vi "mqttClient_ModelController.vi"() -> ()   [LabVIEW 2019]
uses:
  state -- cluster.ctl
  <vilib>/LabVIEW Open Source Project/OpenSerializer JKI JSON/Serializer.JSON.lvclass
  C:/Program Files (x86)/National Instruments/LabVIEW 2019/vi.lib/LabVIEW Open Source Project/OpenSerializer/Serializer/Serializer.lvclass
  target -- cluster.ctl
  <vilib>/LabVIEW Open Source Project/MQTT Connection/MQTT_Base/Base Class/MQTT_Base.lvclass/MQTT_Base.ctl
  <vilib>/LabVIEW Open Source Project/MQTT Client/Client class/Client.lvclass/Client.ctl
  <vilib>/LabVIEW Open Source Project/MQTT Control Packets/Control Packets/ControlPacket/QualityOfService -- enum.ctl
  <vilib>/LabVIEW Open Source Project/MQTT Control Packets/Control Packets/ControlPacket/ControlPacket.lvclass/ControlPacket.ctl
  <vilib>/LabVIEW Open Source Project/MQTT Control Packets/Control Packets/CONNECT/ConnectFlags -- cluster.ctl
  <vilib>/LabVIEW Open Source Project/MQTT TCP Connection/MQTT_TCP/Connection/TCPConnection.lvclass
  C:/Program Files (x86)/National Instruments/LabVIEW 2019/vi.lib/LabVIEW Open Source Project/MQTT Connection/MQTT_Connection/Connection/Connection.lvclass
  <vilib>/LabVIEW Open Source Project/MQTT Client/Client class/Client.lvclass
  C:/Program Files (x86)/National Instruments/LabVIEW 2019/vi.lib/LabVIEW Open Source Project/MQTT Connection/MQTT_Base/Base Class/MQTT_Base.lvclass
  <vilib>/LabVIEW Open Source Project/OpenSerializer/Serializer.FlattenedString/Serializer.FlattenedString.lvclass
  <vilib>/LabVIEW Open Source Project/MQTT Control Packets/Control Packets/PUBLISH/PUBLISH.lvclass
  C:/Program Files (x86)/National Instruments/LabVIEW 2019/vi.lib/LabVIEW Open Source Project/MQTT Control Packets/Control Packets/ControlPacket/ControlPacket.lvclass
  <vilib>/LabVIEW Open Source Project/OpenSerializer/Serializer/Serializer.lvclass
  <vilib>/numeric/Random Number (Range) DBL.vi
  <vilib>/LabVIEW Open Source Project/MQTT Connection/MQTT_Base/Base Class/MQTT_Base.lvclass
  <vilib>/LabVIEW Open Source Project/MQTT Control Packets/Control Packets/ControlPacket/ControlPacket.lvclass
  <vilib>/LabVIEW Open Source Project/MQTT Control Packets/Control Packets/CONNECT/CONNECT.lvclass
panel:
  in  "Connection":bool
  out "Last Error":errorcluster
  out "Incoming Payload":string
  out "state":T1 {"measured" format="%.1g"; "setpoint" format="%.1g"}
  # "Native LabVIEW MQTT Client (Model - Controller)"
  # "G Open Source Project for LabVIEW\nhttps://github.com/LabVIEW-Open-Source/MQTT-Client"
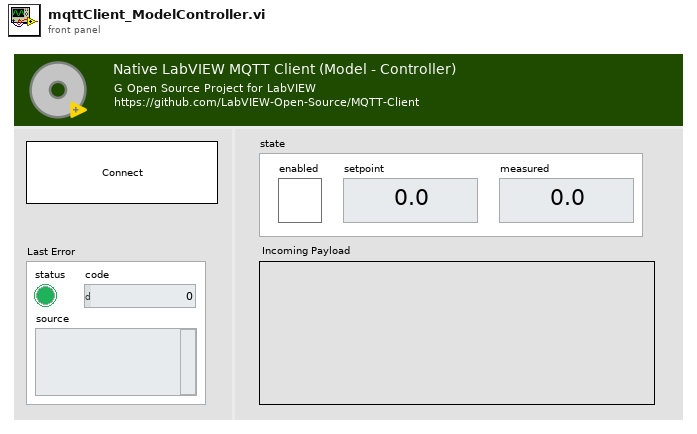
[diagram p1: front panel]
types:
  T1 = typedef "state -- cluster.ctl" = cluster{"enabled":bool, "setpoint":dbl, "measured":dbl}
  T2 = typedef "target -- cluster.ctl" = cluster{"enabled":bool, "setpoint":dbl, "responseURI":string}
  T3 = cluster{"appName":string, "state":T1, "target":T2}
  T4 = typedef "MQTT Client.lvlib/Client.lvclass/Public Events -- cluster.ctl" = cluster{"Connection Status":refnum<user-event>, "Connected":refnum<user-event>, "Application Message":refnum<user-event>}
  T5 = typedef "MQTT Base.lvlib/MQTT_Base.lvclass/Public Events -- cluster.ctl" = cluster{"Stop Event":refnum<user-event>, "Error Event":refnum<user-event>, "Inbound Message":refnum<user-event>}
  T6 = typedef "MQTT_Control_Packets.lvlib/ControlPacket.lvclass/QualityOfService -- enum.ctl" = enum16{"0 (At Most Once)", "1 (At Least Once)", "2 (Exactly Once)"}
  T7 = typedef "MQTT_Control_Packets.lvlib/CONNECT.lvclass/ConnectFlags -- cluster.ctl" = cluster{"Reserved":bool, "Clean Session":bool, "Will Flag":bool, "Will QoS 1":bool, "Will QoS 2":bool, "Will Retain":bool, "Password Flag":bool, "User Name Flag":bool}
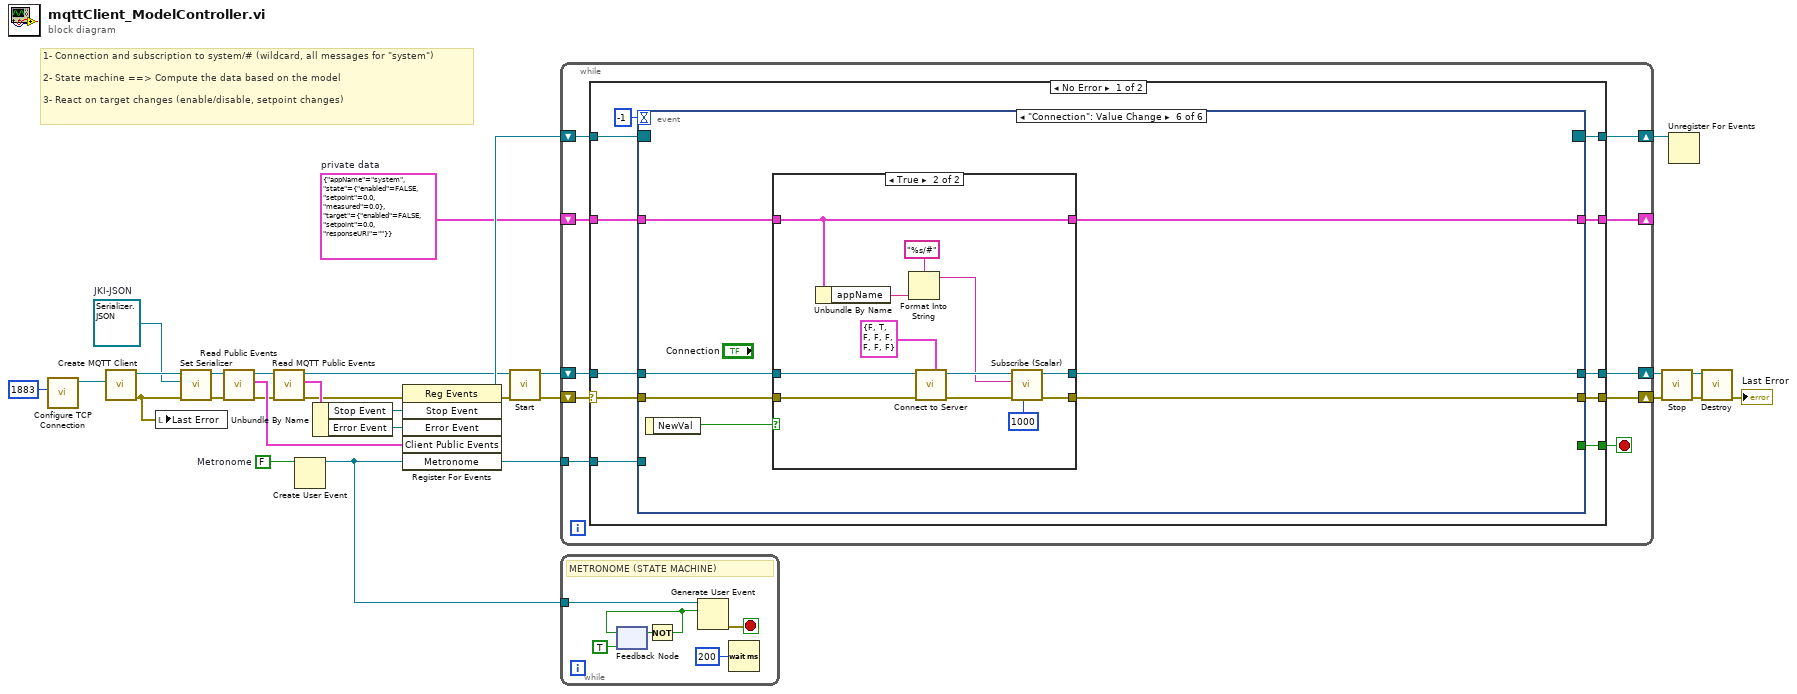
[diagram p0: block diagram]
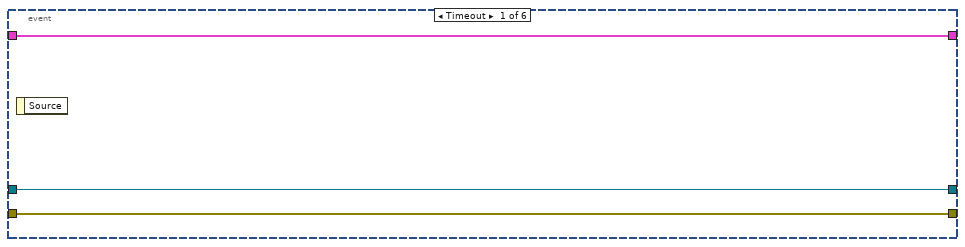
[diagram p2: hidden frame]
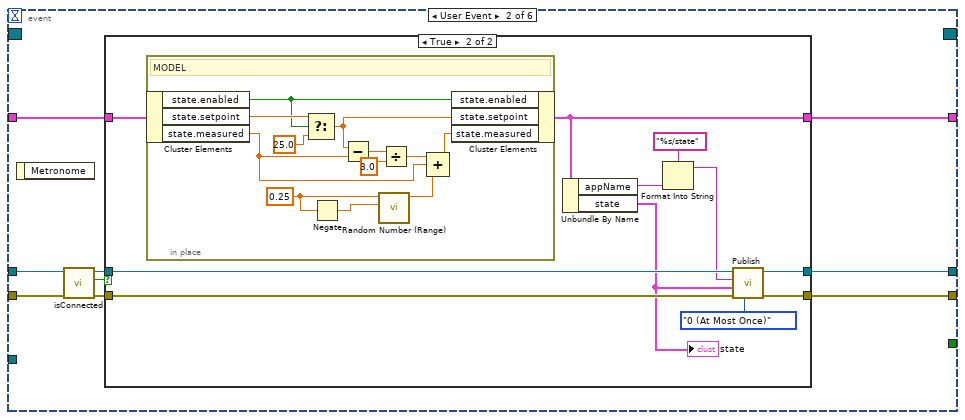
[diagram p3: hidden frame]
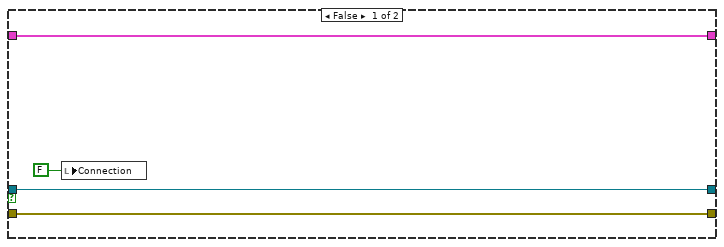
[diagram p4: hidden frame]
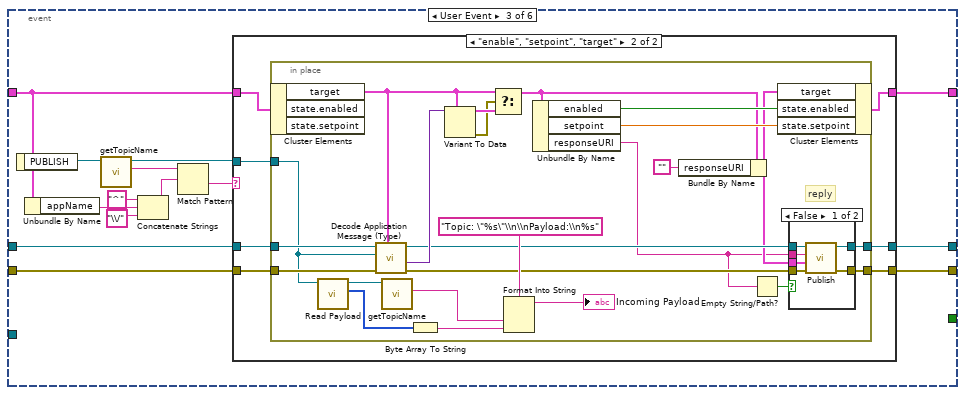
[diagram p5: hidden frame]
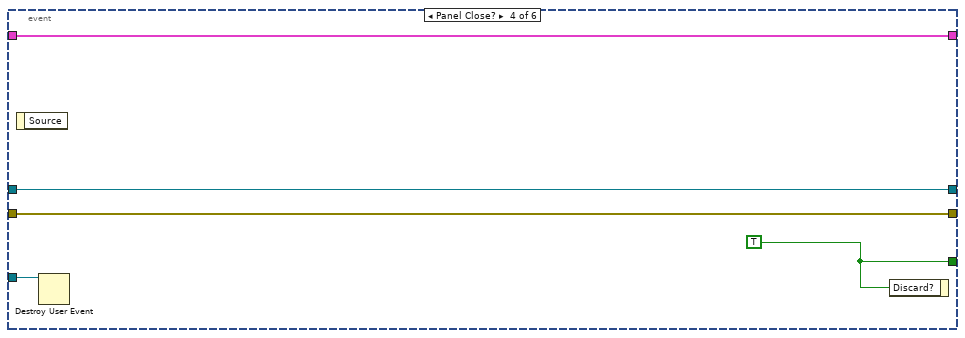
[diagram p8: hidden frame]
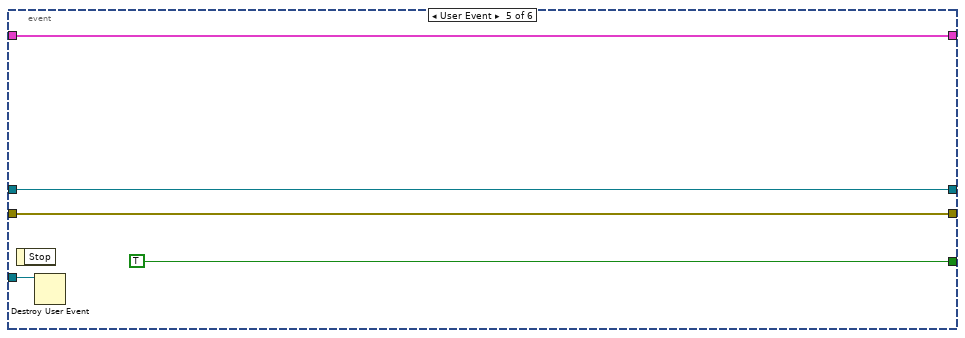
[diagram p9: hidden frame]
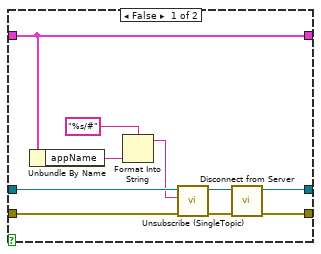
[diagram p10: hidden frame]
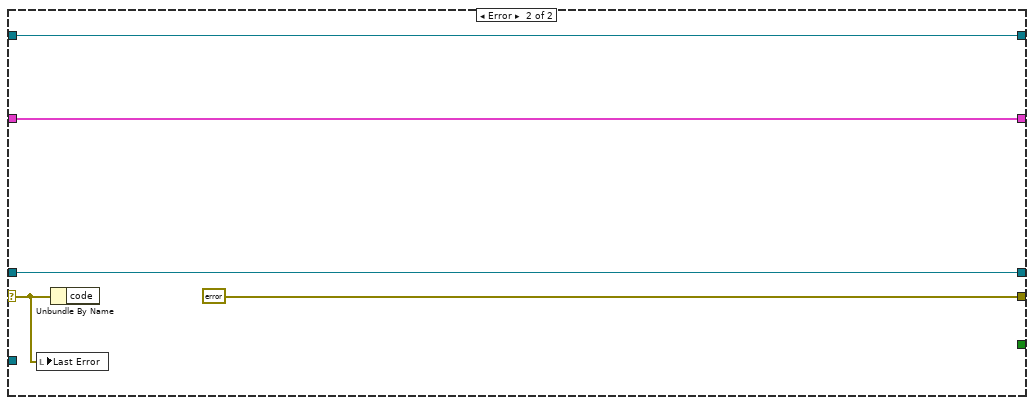
[diagram p11: hidden frame]
diagram:
  w2 = FALSE  # Metronome
  w4 = T3 {"appName"="system", "state"={"enabled"=FALSE, "setpoint"=0.0, "measured"=0.0}, "target"={"enabled"=FALSE, "setpoint"=0.0, "responseURI"=""}}  # private data
  w7 = refnum<class "Serializer.JSON.lvclass"> refnum  # JKI-JSON
  # "1- Connection and subscription to system/# (wildcard, all messages for \"system\")\n\n2- State machine ==> Compute the data based on the model\n\n3- React on target changes (enable/disable, setpoint changes)"
  n1 = call <vilib>:"Configure TCP Connection.vi"("remote port (80)"=u16 1883) -> ("TCPConnection"=w11:refnum<class "TCPConnection.lvclass">)  [unwired: 9 in, 1 out]
  n2 = call <vilib>:"Create MQTT Client.vi"("Connection Configuration"=w11) -> ("error out"=w3:errorcluster, "Client out"=w10:refnum<class "Client.lvclass">)  [unwired: 9 in]
  n3 = local write "Last Error"(w3) -> ()
  n4 = call <vilib>:"Set Serializer.vi"("error in (no error)"=w3, "Serializer (default: Flattened String)"=w7, "MQTT_Base"=w10) -> ("error out"=w8:errorcluster, "MQTT_Base out"=w9:refnum<class "Client.lvclass">)  [unwired: 7 in]
  n5 = call <vilib>:"Read Public Events.vi"("error in (no error)"=w8, "Client in"=w9) -> ("error out"=w13:errorcluster, "Client Public Events"=w15:T4, "Client out"=w12:refnum<class "Client.lvclass">)  [unwired: 7 in]
  n6 = call <vilib>:"Read MQTT Public Events.vi"("error in (no error)"=w13, "MQTT_Base in"=w12) -> ("error out"=w14:errorcluster, "MQTT Public Events"=w22:T5, "MQTT_Base out"=w17:refnum<class "Client.lvclass">)  [unwired: 7 in]
  n7 = Create User Event(user event datatype=w2) -> (user event=w1:refnum<user-event>)  [unwired: 1 in, 1 out]
  n8 = Unbundle By Name(w22) -> ("Stop Event"=w20:refnum<user-event>, "Error Event"=w21:refnum<user-event>)
  n9 = register-events(error in=w14, w20, w21, w15, w1) -> (reference out=w18:refnum<event-registration>, error out=w16:errorcluster)  [unwired: 1 in]
  n10 = call <vilib>:"Start.vi"("error in (no error)"=w16, "MQTT_Base in"=w17) -> ("error out"=w5:errorcluster, "MQTT_Base out"=w6:refnum<class "Client.lvclass">)  [unwired: 7 in, 1 out]
  n11 = while {
    shift-right: [w37] -> w19
    shift-left: w18 -> [w38]
    shift-right: [w34] -> w24
    shift-left: w6 -> [w35]
    shift-right: [w36] -> w26
    shift-left: w5 -> [w32]
    shift-right: [w30] -> _
    shift-left: w4 -> [w31]
    tunnel: w1 -> [w29]
    stop <- w33 stop-if-true
    n12 = case shown="No Error" w32 {
      selector: w32 -> [w42 w187]
      tunnel: w38 -> [w49 w186]
      tunnel: [w48 w186] -> w37
      tunnel: [w47 errorcluster {"status"=FALSE, "code"=0, "source"=""} ("error out")] -> w36
      tunnel: w35 -> [w45 w188]
      tunnel: [w44 w188] -> w34
      tunnel: [w43 _] -> w33
      tunnel: w31 -> [w41 w185]
      tunnel: [w40 w185] -> w30
      tunnel: w29 -> [w39 _]
      frame No Error {
        n13 = event shown="[5] \"Connection\": Value Change" {
          selector: w49 -> [_ _ _ _ _ _]
          dyn-events: [_ _ _ _ _ _] -> w48
          timeout: -1 -> [_ _ _ _ _ _]
          tunnel: w42 -> [w50 w57 w99 w147 w154 w157]
          tunnel: [w50 w60 w97 w147 w154 w158] -> w47
          tunnel: [_ _ _ w149 TRUE _] -> w43
          tunnel: w45 -> [w51 w59 w100 w148 w152 w161]
          tunnel: [w51 w61 w98 w148 w152 w159] -> w44
          tunnel: w41 -> [w52 w54 w95 w146 w151 w155]
          tunnel: [w52 w53 w96 w146 w151 w156] -> w40
          tunnel: w39 -> [_ _ _ w145 w150 _]
          event Timeout {
            n14 = event-data() -> ()  [unwired: 1 in, 1 out]
          }
          event User Event {
            n15 = event-data() -> ()  [unwired: 1 in, 1 out]
            n16 = call <vilib>:"isConnected.vi"("error in (no error)"=w57, "Client in"=w59) -> ("error out"=w56:errorcluster, "connected"=w55:bool, "Client out"=w58:refnum<class "Client.lvclass">)  [unwired: 7 in]
            n17 = case shown="True" w55 {
              tunnel: [w65 w75] -> w61
              tunnel: [w64 w73] -> w60
              tunnel: w58 -> [w65 w76]
              tunnel: w56 -> [w64 w74]
              tunnel: w54 -> [w62 w69]
              tunnel: [w62 w68] -> w53
              frame False {
                n18 = local write "Connection"(FALSE ("Connection")) -> ()
              }
              frame True {
                n19 = in-place {
                  w78 = 0.25 ("lower bound (0)")
                  # "MODEL"
                  n20 = in-place-cluster #1(w69) -> ("state.enabled"=w86:bool, "state.setpoint"=w87:dbl, "state.measured"=w81:dbl)
                  n21 = Select(t=w87, s=w86, f=25.0) -> (s? t:f=w85:dbl)
                  n22 = Negate(x=w78) -> (-x=w79:dbl)
                  n23 = Subtract(x=w85, y=w81) -> (x-y=w83:dbl)
                  n24 = call-poly <vilib>:"Random Number (Range).vi"("lower bound (0)"=w79, "upper bound (100)"=w78) -> ("number"=w77:dbl)  [unwired: 9 in]
                  n25 = Divide(x=w83, y=3.0 ("f")) -> (x/y=w82:dbl)
                  n26 = Compound Arithmetic op=ADD(w82, w81, w77) -> (w80:dbl)
                  n27 = in-place-cluster #1("state.enabled"=w86, "state.setpoint"=w85, "state.measured"=w80) -> (w68:T3)
                }
                n28 = Unbundle By Name(w68) -> ("appName"=w66:string, "state"=w67:T1)
                "state" <- w67
                n29 = Format Into String(format string="%s/state" ("Topic Name (empty: Payload name)"), w66) -> (resulting string=w70:string)  [unwired: 2 in, 1 out]
                n30 = call <vilib>:"Publish.vi"("QoS"=QualityOfService_--_enum."0 (At Most Once)", "error in (no error)"=w74, "Payload"=w67, "Topic Name (empty: Payload name)"=w70, "Client in"=w76) -> ("error out"=w73:errorcluster, "Client out"=w75:refnum<class "Client.lvclass">)  [unwired: 4 in, 1 out]
              }
            }
          }
          event User Event {
            n31 = event-data() -> ("PUBLISH"=w102:refnum<class "PUBLISH.lvclass">)  [unwired: 1 in]
            n32 = Unbundle By Name(w95) -> ("appName"=w94:string)
            n33 = call <vilib>:"getTopicName.vi"("PUBLISH in"=w102) -> ("Topic"=w90:string, "PUBLISH out"=w101:refnum<class "PUBLISH.lvclass">)  [unwired: 8 in, 1 out]
            n34 = Concatenate Strings("^" ("string"), w94, "\\/" ("string")) -> (w91:string)
            n35 = Match Pattern(string=w90, regular expression=w91) -> (after substring=w89:string)  [unwired: 1 in, 3 out]
            n36 = case shown="\"enable\", \"setpoint\", \"target\"" w89 {
              tunnel: w101 -> [_ w108]
              tunnel: w100 -> [w105 w110]
              tunnel: w99 -> [w104 w109]
              tunnel: [w105 w107] -> w98
              tunnel: [w104 w106] -> w97
              tunnel: w95 -> [w103 w112]
              tunnel: [w103 w111] -> w96
              frame Default {
              }
              frame "enable", "setpoint", "target" {
                n37 = in-place {
                  in-place-border: w110 -> [w136]
                  in-place-border: w109 -> [w135]
                  in-place-border: w108 -> [w131]
                  in-place-border: [w118] -> w107
                  in-place-border: [w120] -> w106
                  # "reply"
                  n38 = in-place-cluster #2(w112) -> ("target"=w132:T2)  [unwired: 2 out]
                  n39 = call <vilib>:"Read Payload.vi"("ControlPacket in"=w131) -> ("Payload"=w130:u8[], "ControlPacket out"=w126:refnum<class "PUBLISH.lvclass">)  [unwired: 9 in]
                  n40 = call <vilib>:"Decode Application Message (Type).vi"("Type"=w132, "error in (no error)"=w135, "PUBLISH"=w131, "Client in"=w136) -> ("error out"=w121:errorcluster, "Payload"=w134:variant, "Client out"=w119:refnum<class "Client.lvclass">)  [unwired: 4 in, 1 out]
                  n41 = call <vilib>:"getTopicName.vi"("PUBLISH in"=w126) -> ("Topic"=w124:string)  [unwired: 8 in, 2 out]
                  n42 = Byte Array To String(unsigned byte array=w130) -> (string=w123:string)
                  n43 = Variant To Data(type=w132, Variant=w134) -> (data=w133:T2, error out=w127:errorcluster)  [unwired: 1 in]
                  n44 = Select(t=w132, s=w127, f=w133) -> (s? t:f=w116:T2)
                  n45 = Format Into String(format string="Topic: \"%s\"\\n\\nPayload:\\n%s", w124, w123) -> (resulting string=→"Incoming Payload":string)  [unwired: 2 in, 1 out]
                  n46 = Unbundle By Name(w116) -> ("enabled"=w129:bool, "setpoint"=w128:dbl, "responseURI"=w113:string)
                  n47 = Bundle By Name(cluster=w116, "responseURI"="") -> (w115:T2)
                  n48 = Empty String/Path?(string/path=w113) -> (empty?=w114:bool)
                  n49 = in-place-cluster #2("target"=w115, "state.enabled"=w129, "state.setpoint"=w128) -> (w111:T3)
                  n50 = case shown="False" w114 {
                    tunnel: w121 -> [w142 w143]
                    tunnel: [w141 w143] -> w120
                    tunnel: w119 -> [w140 w144]
                    tunnel: [w139 w144] -> w118
                    tunnel: w113 -> [w138 _]
                    tunnel: w115 -> [w137 _]
                    frame False {
                      n51 = call <vilib>:"Publish.vi"("error in (no error)"=w142, "Payload"=w137, "Topic Name (empty: Payload name)"=w138, "Client in"=w140) -> ("error out"=w141:errorcluster, "Client out"=w139:refnum<class "Client.lvclass">)  [unwired: 5 in, 1 out]
                    }
                    frame True {
                    }
                  }
                }
              }
            }
          }
          event Panel Close? {
            w149 = TRUE
            n52 = event-data() -> ()  [unwired: 1 in, 1 out]
            n53 = Destroy User Event(user event=w145) -> ()  [unwired: 1 in, 1 out]
            n54 = event-data("Discard?"=w149) -> ()  [unwired: 1 in, 1 out]
          }
          event User Event {
            n55 = event-data() -> ()  [unwired: 1 in, 1 out]
            n56 = Destroy User Event(user event=w150) -> ()  [unwired: 1 in, 1 out]
          }
          event "Connection": Value Change {
            n57 = event-data() -> ("NewVal"=w160:bool)  [unwired: 1 in]
            n58 = case shown="True" w160 {
              tunnel: w161 -> [w168 w183]
              tunnel: [w171 w176] -> w159
              tunnel: [w170 w178] -> w158
              tunnel: w157 -> [w166 w182]
              tunnel: [w163 w181] -> w156
              tunnel: w155 -> [w163 w181]
              frame False {
                n59 = Unbundle By Name(w163) -> ("appName"=w165:string)
                n60 = Format Into String(format string="%s/#" ("Topic Name (empty: Payload name)"), w165) -> (resulting string=w162:string)  [unwired: 2 in, 1 out]
                n61 = call <vilib>:"Unsubscribe (SingleTopic).vi"("error in (no error)"=w166, "Topic Filter"=w162, "MQTT_Base in"=w168) -> ("error out"=w167:errorcluster, "MQTT_Base out"=w169:refnum<class "Client.lvclass">)  [unwired: 6 in, 1 out]
                n62 = call <vilib>:"Disconnect from Server.vi"("error in (no error)"=w167, "Client in"=w169) -> ("error out"=w170:errorcluster, "Client out"=w171:refnum<class "Client.lvclass">)  [unwired: 7 in, 1 out]
              }
              frame True {
                n63 = Unbundle By Name(w181) -> ("appName"=w174:string)
                n64 = Format Into String(format string="%s/#" ("Topic Name (empty: Payload name)"), w174) -> (resulting string=w172:string)  [unwired: 2 in, 1 out]
                n65 = call <vilib>:"Connect to Server.vi"("Connect Flags"=T7 {"Reserved"=FALSE, "Clean Session"=TRUE, "Will Flag"=FALSE, "Will QoS 1"=FALSE, "Will QoS 2"=FALSE, "Will Retain"=FALSE, "Password Flag"=FALSE, "User Name Flag"=FALSE}, "error in (no error)"=w182, "Client in"=w183) -> ("error out"=w175:errorcluster, "Client out"=w177:refnum<class "Client.lvclass">)  [unwired: 5 in, 2 out]
                n66 = call <vilib>:"Subscribe (Scalar).vi"("timeout (1000ms)"=1000 ("timeout (100ms)"), "error in (no error)"=w175, "Topic Filter"=w172, "Client in"=w177) -> ("error out"=w178:errorcluster, "Client out"=w176:refnum<class "Client.lvclass">)  [unwired: 5 in, 1 out]
              }
            }
          }
        }
      }
      frame Error {
        n67 = local write "Last Error"(w187) -> ()
        n68 = Unbundle By Name(w187) -> ()  [unwired: 1 out]
      }
    }
  }
  n69 = while {
    tunnel: w1 -> [w194]
    stop <- w193 stop-if-true
    # "METRONOME (STATE MACHINE)"
    n70 = feedback #3(TRUE) -> (w191:bool)
    n71 = Not(x=w191) -> (.not. x?=w190:bool)
    n72 = feedback-in #3(w190) -> ()
    n73 = Generate User Event(user event=w194, event data cluster=w190) -> (error out=w193:errorcluster)  [unwired: 2 in, 1 out]
    n74 = Wait (ms)(milliseconds to wait=u32 200) -> ()  [unwired: 1 out]
  }
  n75 = call <vilib>:"Stop.vi"("error in (no error)"=w26, "MQTT_Base in"=w24) -> ("error out"=w25:errorcluster, "MQTT_Base out"=w23:refnum<class "Client.lvclass">)  [unwired: 7 in, 1 out]
  n76 = Unregister For Events(event registration refnum=w19) -> ()  [unwired: 1 in, 1 out]
  n77 = call <vilib>:"Destroy.vi"("error in (no error)"=w25, "MQTT_Base in"=w23) -> ("error out"=→"Last Error":errorcluster)  [unwired: 8 in, 1 out]
